vi "UpdateElement(Single).vi"(7 "Qualified Name":string, 8 "error in (no error)":errorcluster, 9 "Value":string, 10 "Key":string, 11 "ConfigManager.Cache in":refnum<class "ConfigManager.Cache.lvclass">) -> (0 "error out":errorcluster, 3 "ConfigManager.Cache out":refnum<class "ConfigManager.Cache.lvclass">)   [LabVIEW 2013, in "CfgManager.lvlib" / "ConfigManager.Cache.lvclass"]
uses:
  ConfigManager.Cache.lvclass
  ConfigManager.Cache.lvclass/ConfigManager.Cache.ctl
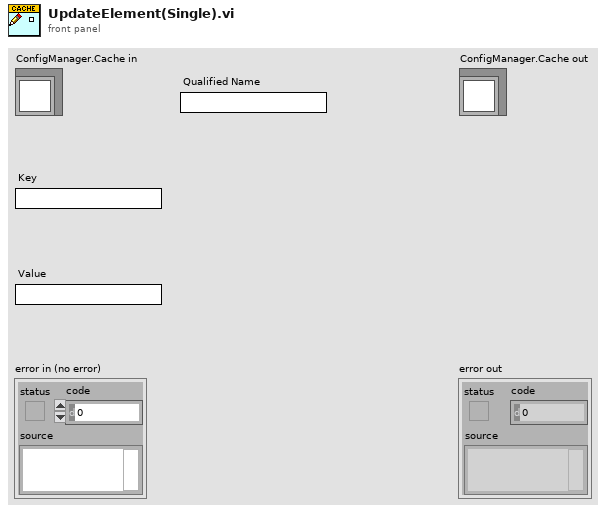
[diagram p1: front panel]
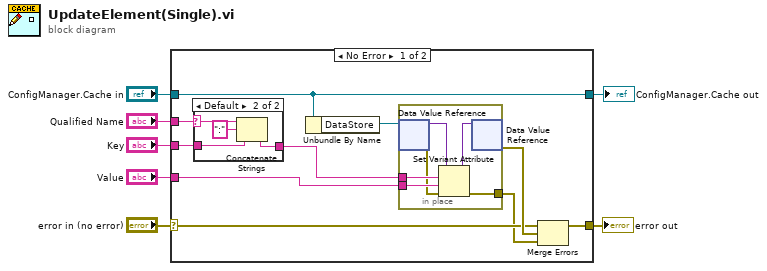
[diagram p0: block diagram]
diagram:
  n1 = case shown="No Error" "error in (no error)" {
    selector: "error in (no error)" -> [w9 w30]
    tunnel: "Value" -> [w17 _]
    tunnel: "Qualified Name" -> [w15 _]
    tunnel: "Key" -> [w14 _]
    tunnel: "ConfigManager.Cache in" -> [w10 w29]
    tunnel: [w11 w30] -> w2
    tunnel: [w10 w29] -> w1
    frame No Error {
      n2 = case shown="Default" w15 {
        selector: w15 -> [_ w19]
        tunnel: w14 -> [w18 w21]
        tunnel: [w18 w20] -> w13
        frame "" {
        }
        frame Default {
          n3 = Concatenate Strings(w19, ":" ("string"), w21) -> (w20:string)
        }
      }
      n4 = Unbundle By Name(w10) -> ("DataStore"=w12:refnum<data-value>)
      n5 = in-place {
        in-place-border: [w28] -> w8
        in-place-border: w13 -> [w27]
        in-place-border: w17 -> [w26]
        n6 = in-place-dvr #1(w12) -> (w23:variant, w25:errorcluster)
        n7 = Set Variant Attribute(Variant=w23, name=w27, value=w26, error in=w25) -> (Variant out=w24:variant, error out=w28:errorcluster)  [unwired: 1 out]
        n8 = in-place-dvr #1(w24) -> (w16:errorcluster)  [unwired: 1 out]
      }
      n9 = Merge Errors(w9, w16, w8) -> (w11:errorcluster)
    }
    frame Error {
    }
  }
  "error out" <- w2
  "ConfigManager.Cache out" <- w1
